vi "Get Group Delay - Fractional Decimator.vi"(10 "sampling rate in":dbl, 11 "output sample rate":fxp<+,48,1>) -> (0 "group delay (s)":dbl format="%#_6p", 2 "sampling rate out":dbl format="%#_6p")   [LabVIEW 2021, in "Digitizer Control.lvclass"]
doc: "Returns the group delay of the fractional decimator in the acquistion path."
uses:
  Digitizer Control.lvclass
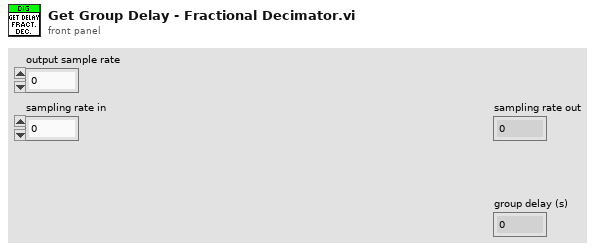
[diagram p1: front panel]
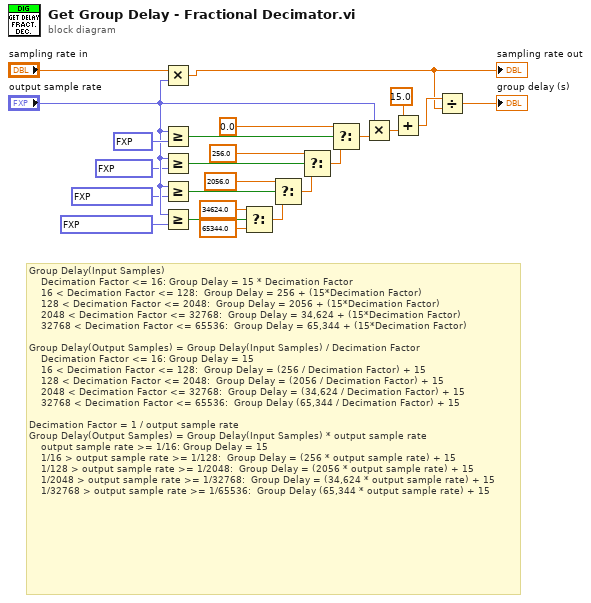
[diagram p0: block diagram]
diagram:
  # "Group Delay(Input Samples)\n    Decimation Factor <= 16: Group Delay = 15 * Decimation Factor\n    16 < Decimation Factor <= 128:  Group Delay = 256 + (15*Decimation Factor)\n    128 < Decimation Factor <= 2048:  Group Delay = 2056 + (15*Decimation Factor)\n    2048 < Decimation Factor <= 32768:  Group Delay = 34,624 + (15*Decimation Factor)\n    32768 < Decimation Factor <= 65536:  Group Delay = 65,344 + (15*Decimation Factor)\n\nGroup Delay(Output Samples) = Group Delay(Input Samples) / Decimation Factor\n    Decimation Factor <= 16: Group Delay = 15 \n    16 < Decimation Factor <= 128:  Group Delay = (256 / Decimation Factor) + 15\n    128 < Decimation Factor <= 2048:  Group Delay = (2056 / Decimation Factor) + 15\n    2048 < Decimation Factor <= 32768:  Group Delay = (34,624 / Decimation Factor) + 15\n    32768 < Decimation Factor <= 65536:  Group Delay (65,344 / Decimation Factor) + 15\n\nDecimation Factor = 1 / output sample rate\nGroup Delay(Output Samples) = Group Delay(Input Samples) * output sample rate\n    output sample rate >= 1/16: Group Delay = 15\n    1/16 > output sample rate >= 1/128:  Group Delay = (256 * output sample rate) + 15\n    1/128 > output sample rate >= 1/2048:  Group Delay = (2056 * output sample rate) + 15\n    1/2048 > output sample rate >= 1/32768:  Group Delay = (34,624 * output sample rate) + 15\n    1/32768 > output sample rate >= 1/65536:  Group Delay (65,344 * output sample rate) + 15"
  n1 = Multiply(x="sampling rate in", y="output sample rate") -> (x*y=w2:dbl)
  "sampling rate out" <- w2
  n2 = Greater Or Equal?(x="output sample rate", y=fxp<+,48,1> 0.0625) -> (x >= y?=w18:bool)
  n3 = Greater Or Equal?(x="output sample rate", y=fxp<+,48,1> 0.0078125) -> (x >= y?=w16:bool)
  n4 = Greater Or Equal?(x="output sample rate", y=fxp<+,48,1> 0.00048828125) -> (x >= y?=w14:bool)
  n5 = Greater Or Equal?(x="output sample rate", y=fxp<+,48,1> 3.0517578125e-05) -> (x >= y?=w11:bool)
  n6 = Select(t=34624.0 ("y"), s=w11, f=65344.0) -> (s? t:f=w9:dbl)
  n7 = Select(t=2056.0 ("y"), s=w14, f=w9) -> (s? t:f=w7:dbl)
  n8 = Select(t=256.0 ("y"), s=w16, f=w7) -> (s? t:f=w5:dbl)
  n9 = Select(t=0.0 ("y"), s=w18, f=w5) -> (s? t:f=w23:dbl)
  n10 = Multiply(x="output sample rate", y=w23) -> (x*y=w21:dbl)
  n11 = Add(x=15.0 ("group delay (decimated samples)"), y=w21) -> (x+y=w3:dbl)
  n12 = Divide(x=w3, y=w2) -> (x/y=→"group delay (s)":dbl)
